vi "Charact One Point.vi"(0 "Scalar SA Path in":refnum<class "SA Abstract Path.lvclass">, 5 "Cal point in":T1, 11 "error in (no error)":errorcluster) -> (4 "Scalar SA Path out":refnum<class "SA Abstract Path.lvclass">, 15 "error out":errorcluster)   [LabVIEW 2023, in "RFFixtureCharact.Public.lvlib" / "SA Abstract Path.lvclass"]
uses:
  SA Abstract Path.lvclass
  C:/srd-semi-rfcal-software/AuxTools/STSRFFixtureCharactUtility/Source/Code Modules/Common/Base Classes/Path/Path.lvclass
  Scalar Path/Type Definitions/Cal Point.ctl
  Scalar Path/Type Definitions/Scalar Charact Result.ctl
  SA Abstract Path.lvclass/SA Abstract Path.ctl
  Properties/Read RFmx Session.vi
  <vilib>/RFmx/SpecAn/mx/RFmxSpecAn.llb/RFmxSpecAn Select Measurement (Single).vi
  <vilib>/RFmx/SpecAn/mx/RFmxSpecAn.llb/RFmxSpecAn TXP Fetch Measurement.vi
  Scalar Path/Scalar Path.lvclass
  RFFixtureCharact.Public.lvlib
  <resource>/objmgr/RFmxSpecAn.rc
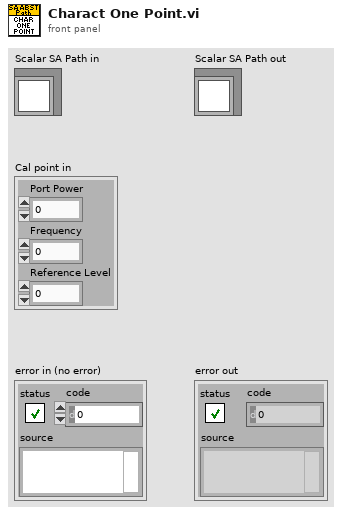
[diagram p1: front panel]
types:
  T1 = typedef "RFFixtureCharact.Public.lvlib/Scalar Path.lvclass/Cal Point.ctl" = cluster{"Port Power":dbl, "Frequency":dbl, "Reference Level":dbl}
  T2 = enum16{"ACP", "CCDF", "CHP", "FCnt", "Harmonics", "OBW", "SEM", "Spectrum", "Spur", "TXP", "AMPM", "DPD", "IQ", "IM", "NF", "PhaseNoise", "PAVT"}
  T3 = typedef "RFFixtureCharact.Public.lvlib/Scalar Path.lvclass/Scalar Charact Result.ctl" = cluster{"Port Power":dbl, "Reference Level":dbl, "Frequency":dbl, "Path Gain":dbl, "Out Of Limit":bool}
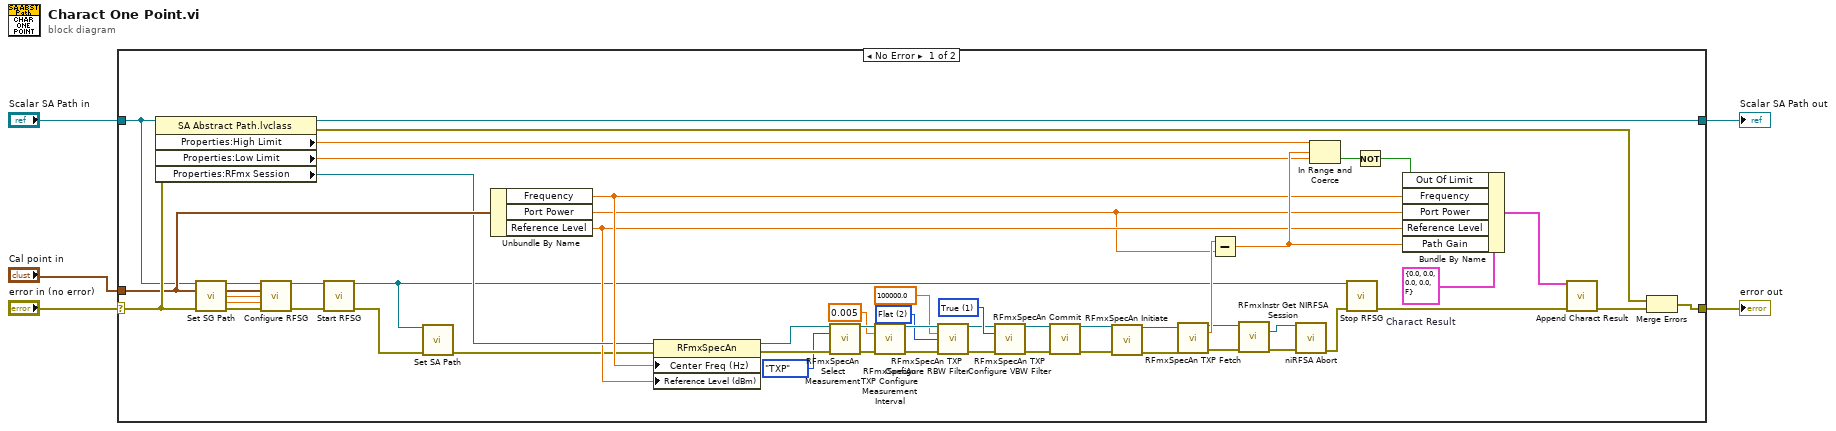
[diagram p0: block diagram]
diagram:
  n1 = case shown="No Error" "error in (no error)" {
    selector: "error in (no error)" -> [w51 w61]
    tunnel: "Scalar SA Path in" -> [w37 w60]
    tunnel: "Cal point in" -> [w49 _]
    tunnel: [w34 w61] -> w2
    tunnel: [w50 w60] -> w3
    frame No Error {
      w10 = 1 items=["False", "True"] ("VBW Auto")
      w12 = 2 items=["None"=5, "Gaussian"=1, "Flat"=2, "RRC"=6] ("RBW Filter Type")
      w57 = T3 {"Port Power"=0.0, "Reference Level"=0.0, "Frequency"=0.0, "Path Gain"=0.0, "Out Of Limit"=FALSE}  # Charact Result
      n2 = property class="SA Abstract Path.lvclass"(reference=w37, error in=w51) -> (reference out=w50:refnum<class "SA Abstract Path.lvclass">, error out=w33:errorcluster, "Properties:High Limit"=w53:dbl, "Properties:Low Limit"=w52:dbl, "Properties:RFmx Session"=w35:refnum<k21>)
      n3 = call-dynamic "Set SG Path.vi"("Path in"=w37, "Cal point in"=w49, "error in (no error)"=w51) -> ("Path out"=w20:refnum<class "SA Abstract Path.lvclass">, "Cal point out"=w21:T1, "Source Gain"=w18:dbl, "Digital Gain"=w30:dbl, "error out"=w19:errorcluster)  [unwired: 8 in]
      n4 = call-dynamic "Configure RFSG.vi"("Path in"=w20, "Cal Point in"=w21, "External Gain"=w18, "Digital Gain"=w30, "error in (no error)"=w19) -> ("Path out"=w58:refnum<class "SA Abstract Path.lvclass">, "error out"=w59:errorcluster)  [unwired: 8 in, 1 out]
      n5 = call-dynamic "Start RFSG.vi"("Path in"=w58, "error in (no error)"=w59) -> ("Path out"=w24:refnum<class "SA Abstract Path.lvclass">, "error out"=w28:errorcluster)  [unwired: 12 in]
      n6 = call-dynamic "Set SA Path.vi"("SA Path in"=w24, "error in (no error)"=w28) -> ("error out"=w27:errorcluster)  [unwired: 12 in, 1 out]
      n7 = Unbundle By Name(w49) -> ("Frequency"=w36:dbl, "Port Power"=w23:dbl, "Reference Level"=w29:dbl)
      n8 = property class="RFmxSpecAn"(reference=w35, error in=w27, "Center Freq (Hz)"=w36, "Reference Level (dBm)"=w29) -> (reference out=w44:refnum<k21>, error out=w45:errorcluster)
      n9 = call-poly <vilib>:"RFmxSpecAn Select Measurement.vi"("Instrument Handle In"=w44, "Measurement"=T2."TXP", "error in (no error)"=w45) -> ("Instrument Handle Out"=w14:refnum<k21>, "error out"=w15:errorcluster)  [unwired: 11 in]
      n10 = call <vilib>:"RFmxSpecAn TXP Configure Measurement Interval.vi"("Instrument Handle In"=w14, "Measurement Interval (s)"=0.005, "error in (no error)"=w15) -> ("Instrument Handle Out"=w17:refnum<k21>, "error out"=w16:errorcluster)  [unwired: 11 in]
      n11 = call <vilib>:"RFmxSpecAn TXP Configure RBW Filter.vi"("Instrument Handle In"=w17, "RBW (Hz)"=100000.0, "RBW Filter Type"=w12, "error in (no error)"=w16) -> ("Instrument Handle Out"=w9:refnum<k21>, "error out"=w7:errorcluster)  [unwired: 10 in]
      n12 = call <vilib>:"RFmxSpecAn TXP Configure VBW Filter.vi"("Instrument Handle In"=w9, "VBW Auto"=w10, "error in (no error)"=w7) -> ("Instrument Handle Out"=w8:refnum<k21>, "error out"=w6:errorcluster)  [unwired: 11 in]
      n13 = call <vilib>:"RFmxSpecAn Commit.vi"("Instrument Handle In"=w8, "error in (no error)"=w6) -> ("Instrument Handle Out"=w40:refnum<k21>, "error out"=w42:errorcluster)  [unwired: 12 in]
      n14 = call <vilib>:"RFmxSpecAn Initiate.vi"("Instrument Handle In"=w40, "error in (no error)"=w42) -> ("Instrument Handle Out"=w39:refnum<k21>, "error out"=w41:errorcluster)  [unwired: 11 in, 1 out]
      n15 = call-poly <vilib>:"RFmxSpecAn TXP Fetch.vi"("Instrument Handle In"=w39, "error in (no error)"=w41) -> ("Instrument Handle Out"=w26:refnum<k21>, "Average Mean Power (dBm)"=w38:dbl, "error out"=w25:errorcluster)  [unwired: 8 in, 3 out]
      n16 = Subtract(x=w38, y=w23) -> (x-y=w54:dbl)
      n17 = call <vilib>:"RFmxInstr Get NIRFSA Session.vi"("Instrument Handle In"=w26, "error in (no error)"=w25) -> ("NI RFSA Session"=w32:refnum<k15>, "error out"=w31:errorcluster)  [unwired: 11 in, 1 out]
      n18 = call <instrlib>:"niRFSA Abort.vi"("instrument handle"=w32, "error in"=w31) -> ("error out"=w22:errorcluster)  [unwired: 12 in, 1 out]
      n19 = In Range and Coerce(upper limit=w53, x=w54, lower limit=w52) -> (In Range?=w55:bool)  [unwired: 1 out]
      n20 = call-dynamic "Stop RFSG.vi"("Path in"=w24, "error in (no error)"=w22) -> ("error out"=w48:errorcluster)  [unwired: 12 in, 1 out]
      n21 = Not(x=w55) -> (.not. x?=w56:bool)
      n22 = Bundle By Name(cluster=w57, "Out Of Limit"=w56, "Frequency"=w36, "Port Power"=w23, "Reference Level"=w29, "Path Gain"=w54) -> (w46:T3)
      n23 = call "Append Charact Result.vi"("Path cal resut in"=w46, "error in (no error)"=w48) -> ("error out"=w47:errorcluster)  [unwired: 13 in]
      n24 = Merge Errors(w33, w47) -> (w34:errorcluster)
    }
    frame Error {
    }
  }
  "error out" <- w2
  "Scalar SA Path out" <- w3
